vi "mod_Kaiser-Bessel Interp FIR design.vi"(2 "Stop Attenuation":dbl format="%.2f", 3 "interpolation factor":i32=1) -> (1 "h":dbl[](array[numeric]) format="%.2f")   [LabVIEW 2020, in "niAMT.lvlib"]
uses:
  <vilib>/addons/Modulation/niAMT.lvlib
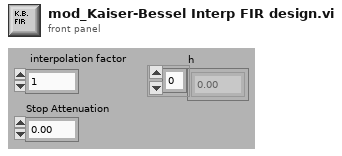
[diagram p1: front panel]
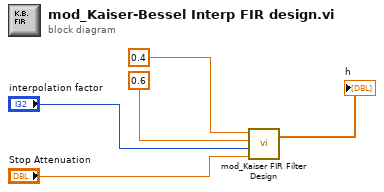
[diagram p0: block diagram]
diagram:
  n1 = call <vilib>:"mod_Kaiser FIR Filter Design.vi"("Stop Attenuation"="Stop Attenuation", "sampling freq: fs"="interpolation factor", "high cutoff freq: fh"=0.6, "low cutoff freq: fl"=0.4) -> ("h"=→"h":dbl[])  [unwired: 1 out]
